vi "FOURIER TRANSLATION-1.vi"() -> ()   [LabVIEW 2018]
uses:
  <vilib>/express/express analysis/Spectral/Block/exnSpectralBlock spectral measurements RMS poly.vi
  <vilib>/express/express analysis/Spectral/Block/exnSpectralBlock spectral measurements RMS DDT.vi
  <vilib>/express/express analysis/Spectral/XNode/ExpressSpectralMeasurementsBlockNode.xnode
panel:
  in  "stop":bool
  out "Waveform Graph":dynamicdata(graph)
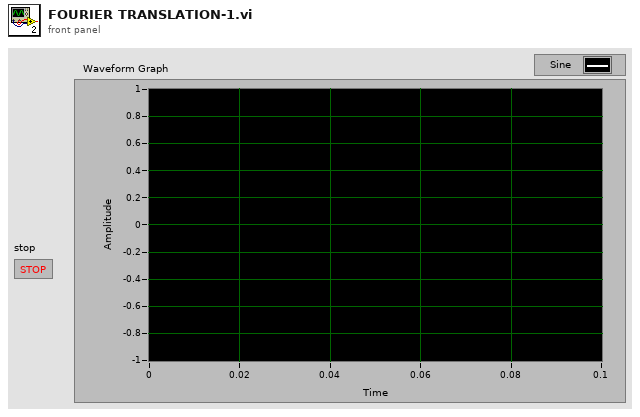
[diagram p1: front panel]
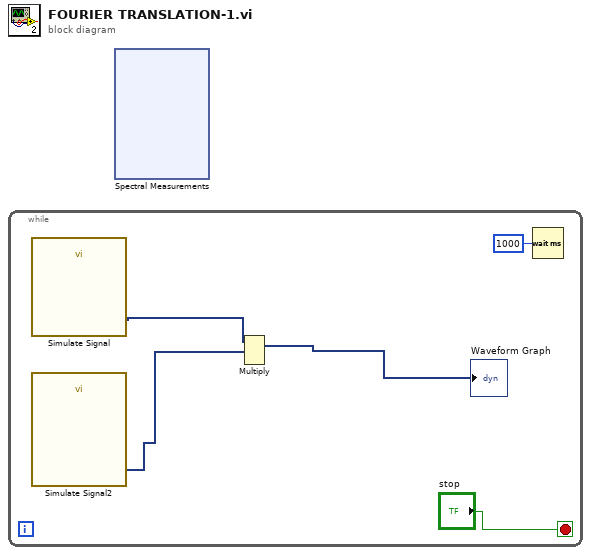
[diagram p0: block diagram]
diagram:
  n1 = while {
    stop <- "stop" stop-if-true
    n2 = call "Simulate Signal"() -> ("Sine"=w2:dynamicdata)  [unwired: 14 in, 1 out]
    n3 = call "Simulate Signal2"() -> ("Sine"=w3:dynamicdata)  [unwired: 14 in, 1 out]
    n4 = Multiply(1:w3, 2:w2) -> (0:→"Waveform Graph":dynamicdata)  [unwired: 1 in, 1 out]
    n5 = Wait (ms)(milliseconds to wait=u32 1000) -> ()  [unwired: 1 out]
  }
  n6 = xnode "Spectral Measurements"() -> ()  [unwired: 2 in, 3 out]
